vi "poly_notify_by_name_single.vi"(8 "error in":errorcluster caption="Error in (no error)", 9 "notifier name":string, 10 "name of caller in (you)":string) -> (0 "error out":errorcluster, 1 "notifier ref out":refnum<vi>, 4 "notified?":bool)   [LabVIEW 2015]
uses:
  ref_tools/polys/poly_control_ref_from_name_caller_single.vi
  ref_tools/ref_tools_eco.vi
  ref_tools/polys/poly_ref_tools_eco_plus.vi
  error_tools/error_handler.vi
  ref_tools/polys/poly_control_ref_from_name_single.vi
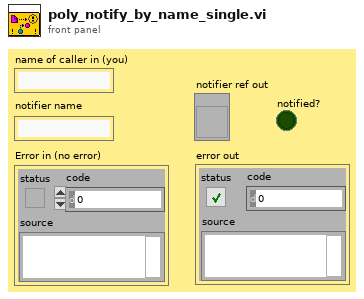
[diagram p1: front panel]
types:
  T1 = typedef "boolean_notifier.ctl" = refnum<notifier>
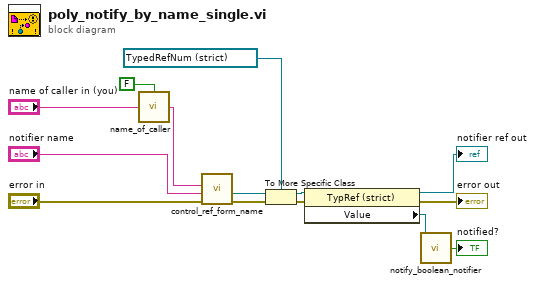
[diagram p0: block diagram]
diagram:
  n1 = call "name_of_caller.vi"("is in inlined vi? (F)"=FALSE, "name of caller in"="name of caller in (you)") -> ("name of caller out"=w4:string)  [unwired: 2 in]
  n2 = call-poly "control_ref_form_name.vi"("error in"="error in", "control name"="notifier name", "name of caller in (your caller)"=w4) -> ("error out"=w8:errorcluster, "control ref"=w14:refnum<vi>)  [unwired: 6 in, 1 out]
  n3 = To More Specific Class(target class=refnum<vi> refnum ("notifier"), reference=w14, error in=w8) -> (specific class reference=w12:refnum<vi>, error out=w7:errorcluster)
  n4 = property class="TypRef (strict)"(reference=w12, error in=w7) -> (reference out=→"notifier ref out":refnum<vi>, error out=→"error out":errorcluster, "Value"=w11:T1)
  n5 = call "notify_boolean_notifier.vi"("TF notifier"=w11) -> ("notified?"=→"notified?":bool)  [unwired: 8 in]
